vi "TiePie.Example.Generator.vi"() -> ()   [LabVIEW 2014, in "LVTiePie.lvlib"]
uses:
  LVTiePie.lvlib
  TiePie.Gen.CfgData.ctl
  TiePie.Gen.handle.ctl
panel:
  out "return type":u8
  out "numberOfListedDevces":u32
  out "GenHandle":T1
  in  "Config":T2={"signal type (sine)"=4, "frequency"=1000.0, "amplitude"=5.0, "offset"=0.0, "Enable"=TRUE} {"signal type (sine)" items=["sine"=1, "triangle"=2, "square"=4, "DC"=8, "noise"=16, "arbitrary"=32, "pulse"=64]}
  in  "symmetry (0-1)":dbl=0.5 format="%#_13g"
  in  "stop":bool
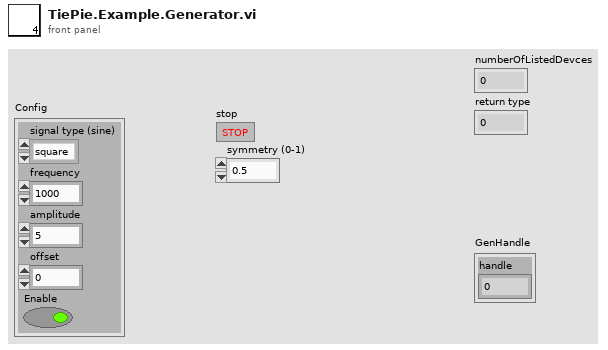
[diagram p1: front panel]
types:
  T1 = typedef "TiePie.Gen.handle.ctl" = cluster{"handle":u32}
  T2 = typedef "TiePie.Gen.CfgData.ctl" = cluster{"signal type (sine)":u32, "frequency":dbl, "amplitude":dbl, "offset":dbl, "Enable":bool}
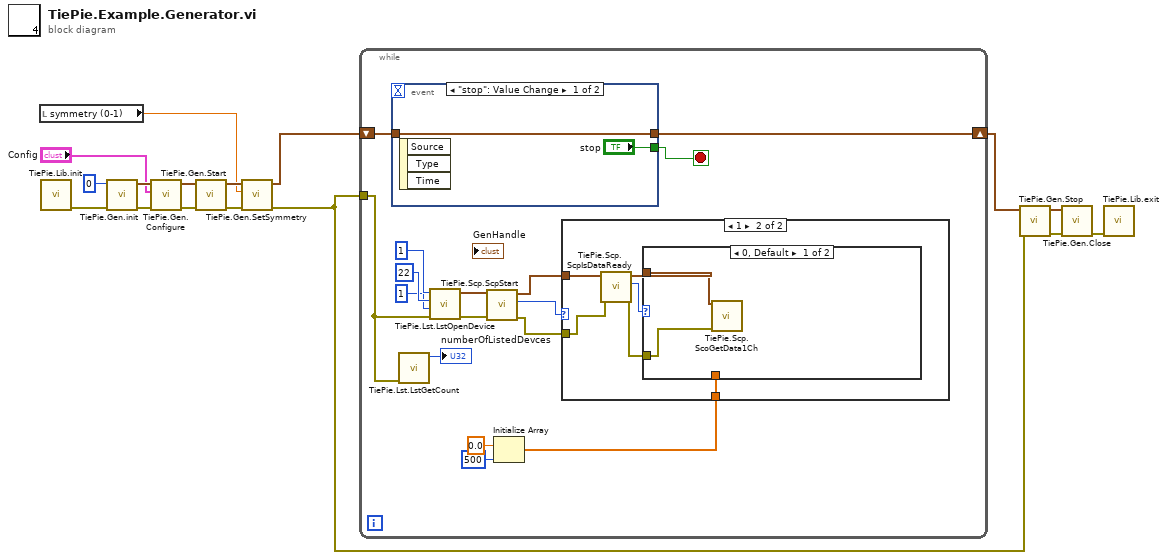
[diagram p0: block diagram]
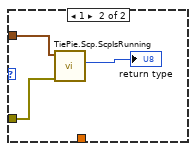
[diagram p3: hidden frame]
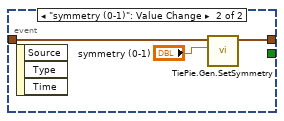
[diagram p4: hidden frame]
diagram:
  n1 = local read "symmetry (0-1)"() -> (w1:dbl)
  n2 = call "TiePie.Lib.init.vi"() -> ("error out"=w15:errorcluster)  [unwired: 11 in]
  n3 = call "TiePie.Gen.init.vi"("error in (no error)"=w15, "DevIndex"=u32 0) -> ("error out"=w14:errorcluster, "GenHandle"=w13:T1)  [unwired: 8 in]
  n4 = call "TiePie.Gen.Configure.vi"("error in (no error)"=w14, "Config"="Config", "GenHandle"=w13) -> ("error out"=w7:errorcluster, "GenHandle out"=w8:T1)  [unwired: 7 in]
  n5 = call "TiePie.Gen.Start.vi"("error in (no error)"=w7, "GenHandle"=w8) -> ("error out"=w5:errorcluster, "GenHandle out"=w3:T1)  [unwired: 8 in]
  n6 = call "TiePie.Gen.SetSymmetry.vi"("error in (no error)"=w5, "symmetry (0-1)"=w1, "GenHandle"=w3) -> ("error out"=w4:errorcluster, "GenHandle out"=w2:T1)  [unwired: 7 in]
  n7 = while {
    tunnel: w4 -> [w26]
    shift-right: [w31] -> w6
    shift-left: w2 -> [w30]
    stop <- w32 stop-if-true
    n8 = event shown="[0] \"stop\": Value Change" {
      selector: _ -> [_ _]
      dyn-events: _ -> [_ _]
      timeout: _ -> [_ _]
      tunnel: ["stop" _] -> w32
      tunnel: w30 -> [w44 w47]
      tunnel: [w44 w46] -> w31
      event "stop": Value Change {
        n9 = event-data() -> ()  [unwired: 1 in, 3 out]
      }
      event "symmetry (0-1)": Value Change {
        n10 = event-data() -> ()  [unwired: 1 in, 3 out]
        n11 = call "TiePie.Gen.SetSymmetry.vi"("symmetry (0-1)"="symmetry (0-1)", "GenHandle"=w47) -> ("GenHandle out"=w46:T1)  [unwired: 8 in, 1 out]
      }
    }
    n12 = call "TiePie.Lst.LstGetCount.vi"("error in (no error)"=w26) -> ("numberOfListedDevces"=→"numberOfListedDevces":u32)  [unwired: 9 in, 1 out]
    n13 = call "TiePie.Lst.LstOpenDevice.vi"("error in (no error)"=w26, "dwDeviceType"=u32 1, "dwId"=u32 22, "dwIdKind"=u32 1) -> ("error out"=w20:errorcluster, "GenHandle"=w21:T1)  [unwired: 6 in]
    n14 = call "TiePie.Scp.ScpStart.vi"("error in (no error)"=w20, "GenHandle"=w21) -> ("error out"=w18:errorcluster, "return type"=w17:u8, "GenHandle out"=w19:T1)  [unwired: 7 in]
    n15 = Initialize Array(0.0 ("element"), 500 ("dimension size")) -> (w22:dbl[])
    n16 = case shown="1" w17 {
      tunnel: w22 -> [_ w35]
      tunnel: w18 -> [_ w33]
      tunnel: w19 -> [_ w34]
      frame 0, Default {
      }
      frame 1 {
        n17 = call "TiePie.Scp.ScpIsDataReady.vi"("error in (no error)"=w33, "GenHandle"=w34) -> ("error out"=w36:errorcluster, "return type"=w38:u8, "GenHandle out"=w37:T1)  [unwired: 7 in]
        n18 = case shown="0, Default" w38 {
          tunnel: w37 -> [w40 w43]
          tunnel: w36 -> [w39 w42]
          tunnel: w35 -> [_ _]
          frame 0, Default {
            n19 = call "TiePie.Scp.ScoGetData1Ch.vi"("GenHandle"=w40, "error in (no error)"=w39) -> ()  [unwired: 11 in, 3 out]
          }
          frame 1 {
            n20 = call "TiePie.Scp.ScpIsRunning.vi"("error in (no error)"=w42, "GenHandle"=w43) -> ("return type"=→"return type":u8)  [unwired: 7 in, 2 out]
          }
        }
      }
    }
  }
  n21 = call "TiePie.Gen.Stop.vi"("error in (no error)"=w4, "GenHandle"=w6) -> ("error out"=w10:errorcluster, "GenHandle out"=w11:T1)  [unwired: 8 in]
  n22 = call "TiePie.Gen.Close.vi"("error in (no error)"=w10, "GenHandle"=w11) -> ("error out"=w9:errorcluster)  [unwired: 9 in]
  n23 = call "TiePie.Lib.exit.vi"("error in (no error)"=w9) -> ()  [unwired: 10 in, 1 out]
